vi "calculateMeanAndStdRobotModel.vi"(8 "error in (no error)":errorcluster, 9 "triples (V0, Vf, V_sent, id)":dbl[][](array[numeric]), 10 "RobotModelArray":T1, 11 "Game in":refnum<class "Game.lvclass">) -> (0 "error out":errorcluster, 1 "Std":T2[](array[typedef]), 2 "Mean":T2[](array[typedef]), 3 "Game out":refnum<class "Game.lvclass">)   [LabVIEW 2023, in "Game.lvclass"]
uses:
  Game.lvclass
  Controls/RobotModel.ctl
  VelocityPlanningTest/Controls/robotModelArray.ctl
  Utilities_class/Utilities.lvclass
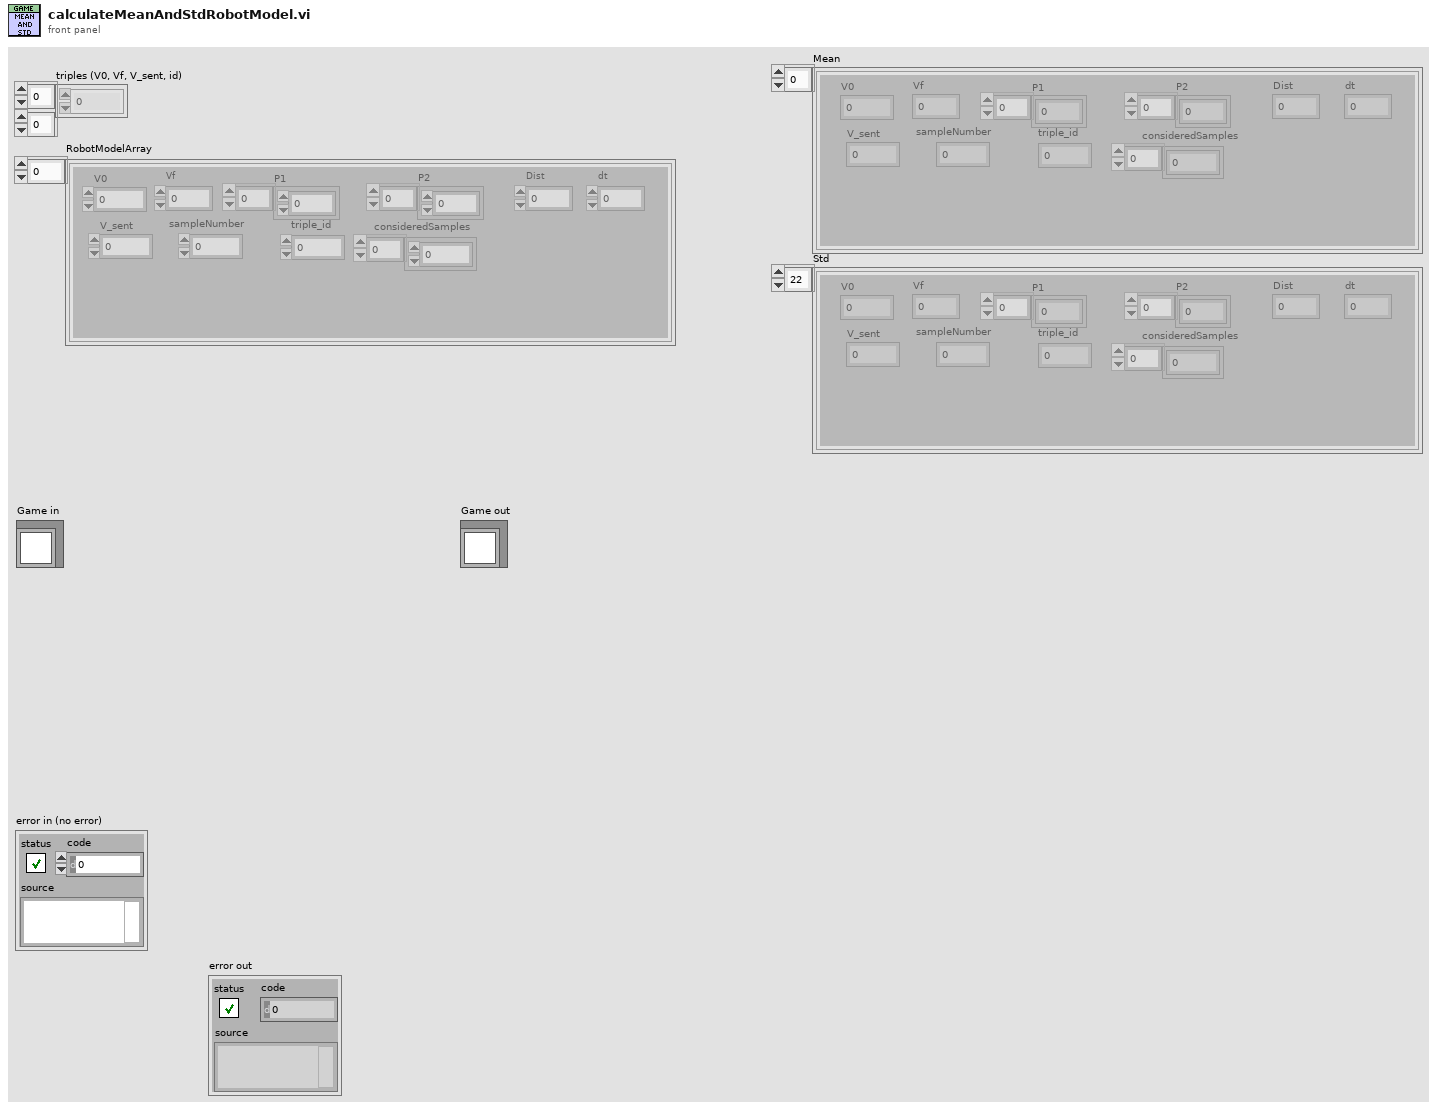
[diagram p1: front panel]
types:
  T1 = typedef "robotModelArray.ctl" = T2[]
  T2 = typedef "RobotModel.ctl" = cluster{"V0":dbl, "Vf":dbl, "Dist":dbl, "dt":dbl, "P1":dbl[], "P2":dbl[], "V_sent":dbl, "sampleNumber":i32, "triple_id":i32, "consideredSamples":dbl[]}
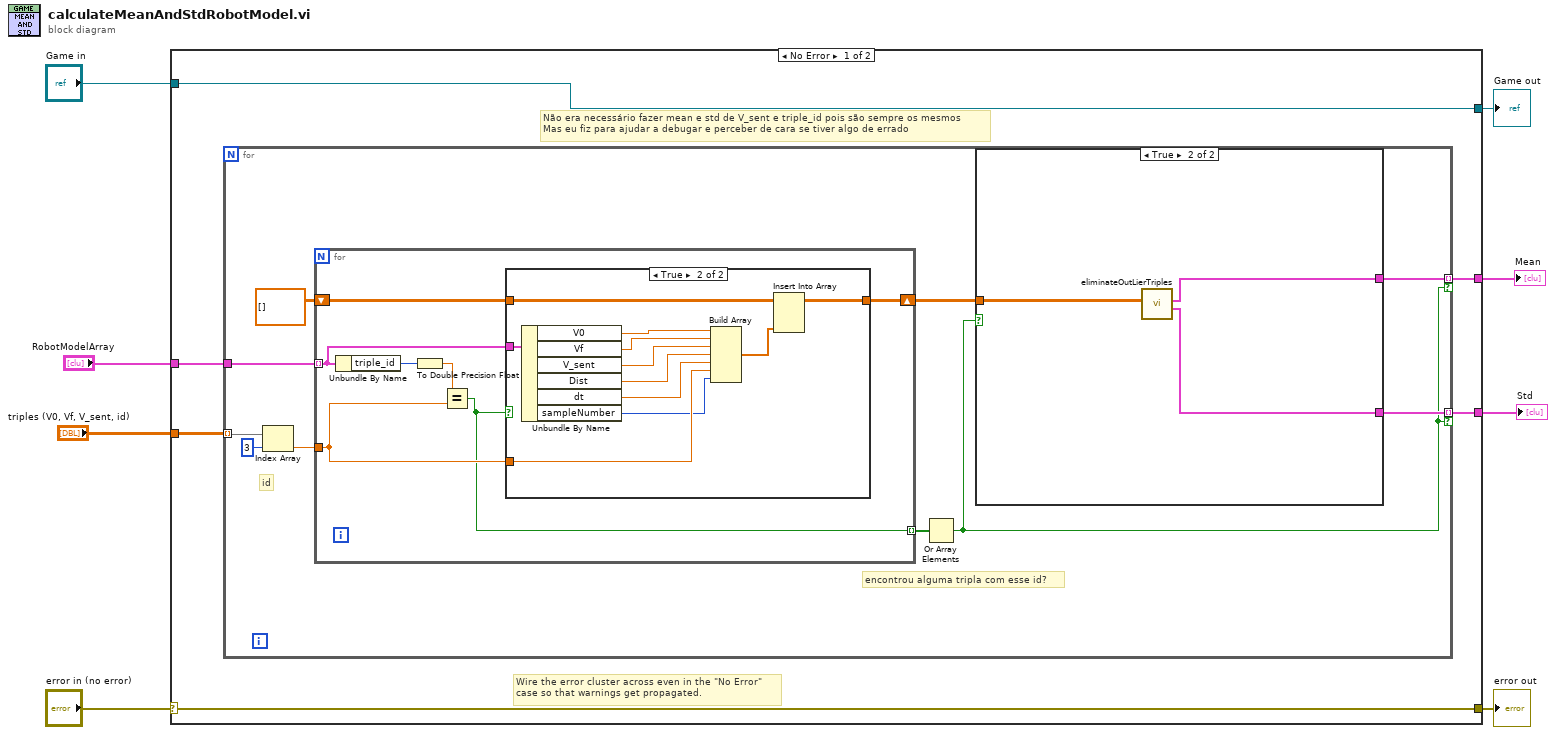
[diagram p0: block diagram]
diagram:
  n1 = case shown="No Error" "error in (no error)" {
    selector: "error in (no error)" -> [w10 w48]
    tunnel: [w10 w48] -> w7
    tunnel: [w14 w47] -> w5
    tunnel: "Game in" -> [w14 w47]
    tunnel: "RobotModelArray" -> [w13 _]
    tunnel: [w12 _] -> w4
    tunnel: [w11 _] -> w3
    tunnel: "triples (V0, Vf, V_sent, id)" -> [w9 _]
    frame No Error {
      # "Não era necessário fazer mean e std de V_sent e triple_id pois são sempre os mesmos\nMas eu fiz para ajudar a debugar e perceber de cara se tiver algo de errado"
      # "Wire the error cluster across even in the \"No Error\"\ncase so that warnings get propagated."
      n2 = for {
        tunnel: w13 -> [w24]
        tunnel: [w21] -> w12 mode=indexing if=w18
        tunnel: [w20] -> w11 mode=indexing if=w18
        tunnel: w9 -> [w17] mode=indexing
        # "id"
        # "encontrou alguma tripla com esse id?"
        n3 = Index Array(array=w17, index=3) -> (element=w15:dbl)
        n4 = for {
          tunnel: w24 -> [w34] mode=indexing
          tunnel: w15 -> [w33]
          shift-right: [w32] -> w22
          shift-left: dbl[][] [] -> [w31]
          tunnel: [w30] -> w19 mode=indexing
          n5 = Unbundle By Name(w34) -> ("triple_id"=w29:i32)
          n6 = To Double Precision Float(number=w29) -> (double precision float=w28:dbl)
          n7 = Equal?(x=w28, y=w33) -> (x = y?=w30:bool)
          n8 = case shown="True" w30 {
            tunnel: w34 -> [_ w46]
            tunnel: w33 -> [_ w40]
            tunnel: [w35 w38] -> w32
            tunnel: w31 -> [w35 w37]
            frame False {
            }
            frame True {
              n9 = Unbundle By Name(w46) -> ("V0"=w45:dbl, "Vf"=w44:dbl, "V_sent"=w43:dbl, "Dist"=w42:dbl, "dt"=w41:dbl, "sampleNumber"=w36:i32)
              n10 = Build Array(w45, w44, w43, w42, w41, w40, w36) -> (w39:dbl[])
              n11 = Insert Into Array(array=w37, new element=w39) -> (w38:dbl[][])  [unwired: 2 in]
            }
          }
        }
        n12 = Or Array Elements(Boolean array=w19) -> (logical OR=w18:bool)
        n13 = case shown="True" w18 {
          tunnel: w22 -> [_ w27]
          tunnel: [_ w26] -> w21
          tunnel: [_ w25] -> w20
          frame False {
          }
          frame True {
            n14 = call "eliminateOutLierTriples.vi"("triplesWith\nSomeId"=w27) -> ("std"=w25:T2, "mean"=w26:T2)  [unwired: 7 in, 2 out]
          }
        }
      }
    }
    frame Error {
    }
  }
  "error out" <- w7
  "Game out" <- w5
  "Mean" <- w4
  "Std" <- w3
